vi "CRYPlot OnOff.vi"(11 "Mouse Point":T1) -> (0 "Invisible Row":i32[](array[numeric]), 1 "Visible Row":i32[](array[numeric]), 2 "Visible?":bool, 3 "Click State?":bool)   [LabVIEW 2013]
uses:
  <vilib>/Utility/miscctls.llb/LVPoint32TypeDef.ctl
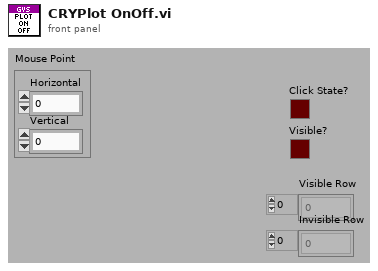
[diagram p1: front panel]
types:
  T1 = typedef "LVPoint32TypeDef.ctl" = cluster{"Horizontal":i32, "Vertical":i32}
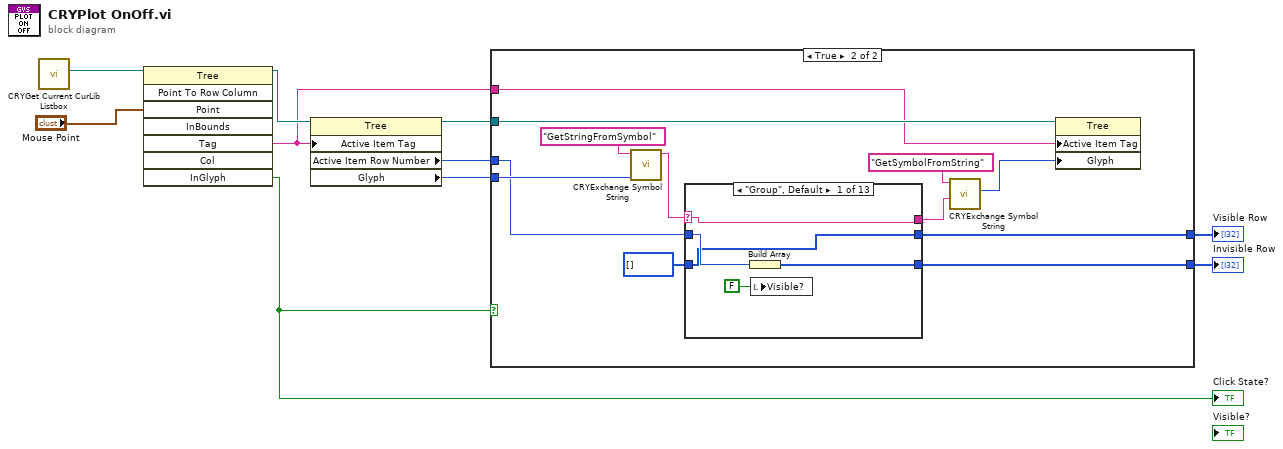
[diagram p0: block diagram]
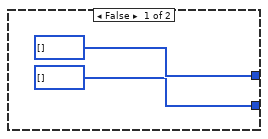
[diagram p2: hidden frame]
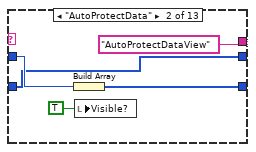
[diagram p3: hidden frame]
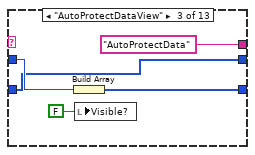
[diagram p4: hidden frame]
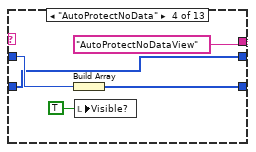
[diagram p5: hidden frame]
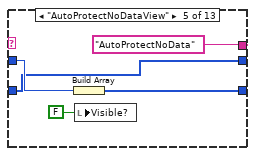
[diagram p6: hidden frame]
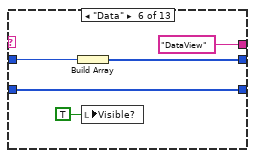
[diagram p7: hidden frame]
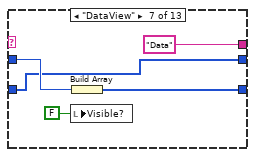
[diagram p8: hidden frame]
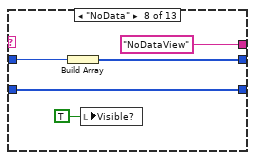
[diagram p9: hidden frame]
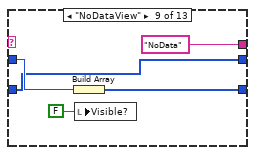
[diagram p10: hidden frame]
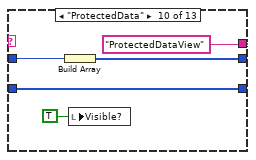
[diagram p11: hidden frame]
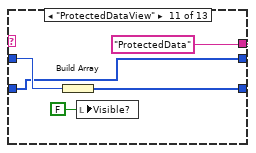
[diagram p12: hidden frame]
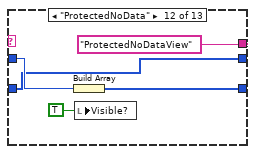
[diagram p13: hidden frame]
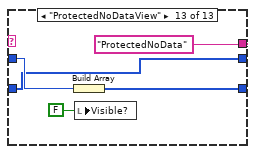
[diagram p14: hidden frame]
diagram:
  n1 = call "CRYGet Current CurLib Listbox.vi"() -> ("CurLib Tree"=w8:refnum<vi>)  [unwired: 9 in, 2 out]
  n2 = invoke on="Invoke Node" class="Tree" method="Point To Row Column"(reference=w8, "Point"="Mouse Point") -> (reference out=w5:refnum<vi>, "Tag"=w2:string, "InGlyph"=w1:bool)  [unwired: 6 in, 5 out]
  "Click State?" <- w1
  n3 = property class="Tree"(reference=w5, "Active Item Tag"=w2) -> (reference out=w4:refnum<vi>, "Active Item Row Number"=w6:i32, "Glyph"=w3:i32)  [unwired: 1 in, 1 out]
  n4 = case shown="True" w1 {
    tunnel: w6 -> [_ w19]
    tunnel: w4 -> [_ w24]
    tunnel: [i32[] [] ("Visible Row") w14] -> w10
    tunnel: [i32[] [] ("Visible Row") w13] -> w9
    tunnel: w3 -> [_ w22]
    tunnel: w2 -> [_ w23]
    frame False {
    }
    frame True {
      n5 = call "CRYExchange Symbol String.vi"("nData"=w22, "sAction"="GetStringFromSymbol") -> ("sData out"=w20:string)  [unwired: 8 in, 1 out]
      n6 = case shown="\"Group\", Default" w20 {
        selector: w20 -> [w25 _ _ _ _ _ _ _ _ _ _ _ _]
        tunnel: [w25 "AutoProtectDataView" ("sData out") "AutoProtectData" ("sData out") "AutoProtectNoDataView" ("sData out") "AutoProtectNoData" ("sData out") "DataView" ("sData out") "Data" ("sData out") "NoDataView" ("sData out") "NoData" ("sData out") "ProtectedDataView" ("sData out") "ProtectedData" ("sData out") "ProtectedNoDataView" ("sData out") "ProtectedNoData" ("sData out")] -> w16
        tunnel: [w26 w31 w36 w41 w46 w53 w56 w63 w66 w73 w76 w81 w86] -> w14
        tunnel: w19 -> [w29 w34 w39 w44 w49 w54 w59 w64 w69 w74 w79 w84 w89]
        tunnel: [w28 w33 w38 w43 w48 w51 w58 w61 w68 w71 w78 w83 w88] -> w13
        tunnel: i32[] [] ("Visible Row") -> [w26 w31 w36 w41 w46 w51 w56 w61 w66 w71 w76 w81 w86]
        frame "Group", Default {
          n7 = Build Array(w29) -> (w28:i32[])
          n8 = local write "Visible?"(FALSE ("Visible?")) -> ()
        }
        frame "AutoProtectData" {
          n9 = Build Array(w34) -> (w33:i32[])
          n10 = local write "Visible?"(TRUE ("Visible?")) -> ()
        }
        frame "AutoProtectDataView" {
          n11 = Build Array(w39) -> (w38:i32[])
          n12 = local write "Visible?"(FALSE ("Visible?")) -> ()
        }
        frame "AutoProtectNoData" {
          n13 = Build Array(w44) -> (w43:i32[])
          n14 = local write "Visible?"(TRUE ("Visible?")) -> ()
        }
        frame "AutoProtectNoDataView" {
          n15 = Build Array(w49) -> (w48:i32[])
          n16 = local write "Visible?"(FALSE ("Visible?")) -> ()
        }
        frame "Data" {
          n17 = Build Array(w54) -> (w53:i32[])
          n18 = local write "Visible?"(TRUE ("Visible?")) -> ()
        }
        frame "DataView" {
          n19 = local write "Visible?"(FALSE ("Visible?")) -> ()
          n20 = Build Array(w59) -> (w58:i32[])
        }
        frame "NoData" {
          n21 = Build Array(w64) -> (w63:i32[])
          n22 = local write "Visible?"(TRUE ("Visible?")) -> ()
        }
        frame "NoDataView" {
          n23 = Build Array(w69) -> (w68:i32[])
          n24 = local write "Visible?"(FALSE ("Visible?")) -> ()
        }
        frame "ProtectedData" {
          n25 = Build Array(w74) -> (w73:i32[])
          n26 = local write "Visible?"(TRUE ("Visible?")) -> ()
        }
        frame "ProtectedDataView" {
          n27 = Build Array(w79) -> (w78:i32[])
          n28 = local write "Visible?"(FALSE ("Visible?")) -> ()
        }
        frame "ProtectedNoData" {
          n29 = Build Array(w84) -> (w83:i32[])
          n30 = local write "Visible?"(TRUE ("Visible?")) -> ()
        }
        frame "ProtectedNoDataView" {
          n31 = Build Array(w89) -> (w88:i32[])
          n32 = local write "Visible?"(FALSE ("Visible?")) -> ()
        }
      }
      n33 = call "CRYExchange Symbol String.vi"("sData"=w16, "sAction"="GetSymbolFromString") -> ("nData out"=w15:i32)  [unwired: 8 in, 1 out]
      n34 = property class="Tree"(reference=w24, "Active Item Tag"=w23, "Glyph"=w15) -> ()  [unwired: 1 in, 2 out]
    }
  }
  "Visible Row" <- w10
  "Invisible Row" <- w9
